vi "Evaluation.vi"(9 "Criteria":enum16{"Less than", "Greater than"}(ring), 10 "Evaluation Threshold":dbl, 11 "Number to Evaluate":dbl) -> (2 "Pass Criteria":bool)   [LabVIEW 2016]
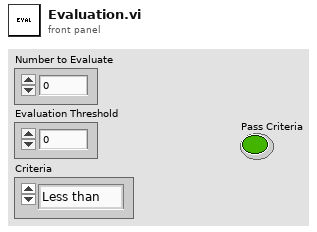
[diagram p1: front panel]
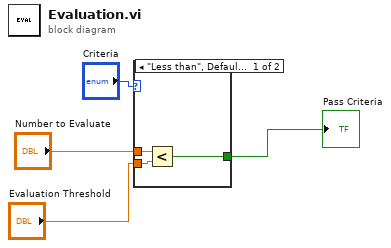
[diagram p0: block diagram]
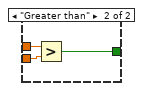
[diagram p2: hidden frame]
diagram:
  n1 = case shown="\"Less than\", Default" "Criteria" {
    tunnel: "Number to Evaluate" -> [w7 w10]
    tunnel: "Evaluation Threshold" -> [w6 w9]
    tunnel: [w5 w8] -> w1
    frame "Less than", Default {
      n2 = Less?(x=w7, y=w6) -> (x < y?=w5:bool)
    }
    frame "Greater than" {
      n3 = Greater?(x=w10, y=w9) -> (0:w8:bool)
    }
  }
  "Pass Criteria" <- w1
